vi "Logger.vi"(8 "wfm data stream":T1, 11 "file path tag":T2) -> (0 "done":bool=TRUE)   [LabVIEW 2023]
uses:
  <extravilib>/ChannelInstances/Tag-path/))Channel.ctl
  <extravilib>/ChannelInstances/Stream-a[.](wfm(dbl))/)Channel.ctl
  <extravilib>/ChannelInstances/Stream-a[.](wfm(dbl))/EndpointRead.vi
  <extravilib>/ChannelInstances/Stream-a[.](wfm(dbl))/)Channel.vi
  <resource>/ChannelSupport/_ChannelSupport/WaitIfNeeded.vi
  <extravilib>/ChannelInstances/Tag-path/EndpointRead.vi
  <vilib>/Waveform/WDTFileIO.llb/Write Waveforms to File (1D).vi
  <extravilib>/ChannelInstances/Tag-path.lvlib
  <extravilib>/ChannelInstances/Stream-a[.](wfm(dbl)).lvlib
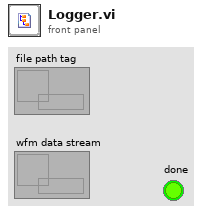
[diagram p1: front panel]
types:
  T1 = typedef "Stream-a[.](wfm(dbl)).lvlib/)Channel.ctl" = refnum<queue>
  T2 = typedef "Tag-path.lvlib/))Channel.ctl" = refnum<queue>
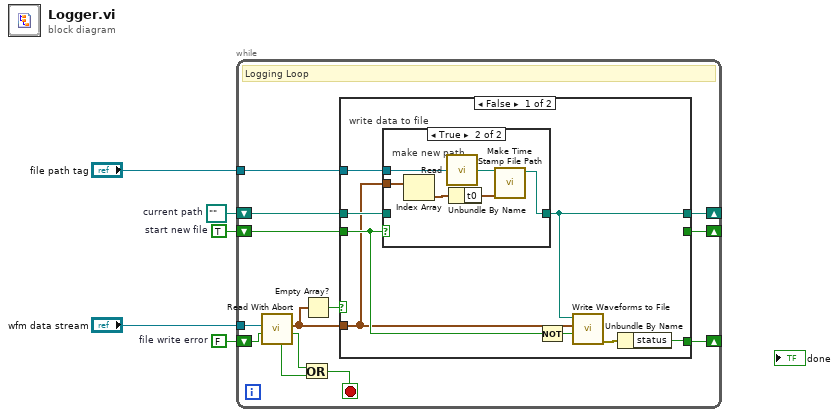
[diagram p0: block diagram]
diagram:
  w5 = FALSE  # file write error
  w4 = path ""  # current path
  w3 = TRUE  # start new file
  n1 = while {
    tunnel: "wfm data stream" -> [w18]
    tunnel: "file path tag" -> [w13]
    shift-right: [w15] -> _
    shift-left: w3 -> [w14]
    shift-right: [w12] -> _
    shift-left: w4 -> [w11]
    shift-right: [w9] -> _
    shift-left: w5 -> [w8]
    stop <- w6 stop-if-true
    # "Logging Loop"
    n2 = call <extravilib>:"Read With Abort.vi"("abort"=w8, "channel"=w18) -> ("last element?"=w16:bool, "element"=w17:waveform(dbl)[], "aborted?"=w7:bool)  [unwired: 4 in, 3 out]
    n3 = Or(x=w16, y=w7) -> (x .or. y?=w6:bool)
    n4 = Empty Array?(array=w17) -> (empty?=w10:bool)
    n5 = case shown="False" w10 {
      selector: w10 -> [_ w34]
      tunnel: w17 -> [w21 _]
      tunnel: [_ w34] -> w15
      tunnel: w14 -> [w22 _]
      tunnel: w13 -> [w25 _]
      tunnel: [w23 _] -> w12
      tunnel: w11 -> [w24 _]
      tunnel: [w19 _] -> w9
      frame False {
        # "write data to file"
        n6 = case shown="True" w22 {
          tunnel: w25 -> [_ w33]
          tunnel: w21 -> [_ w30]
          tunnel: [w27 w32] -> w23
          tunnel: w24 -> [w27 _]
          frame False {
          }
          frame True {
            # "make new path"
            n7 = Index Array(array=w30) -> (element=w31:waveform(dbl))  [unwired: 1 in]
            n8 = call <extravilib>:"Read.vi"("channel"=w33) -> ("element"=w29:path)  [unwired: 1 in, 1 out]
            n9 = Unbundle By Name(w31) -> ("t0"=w28:timestamp)
            n10 = call "Make Time Stamp File Path.vi"("t0"=w28, "base path"=w29) -> ("file path"=w32:path)  [unwired: 9 in]
          }
        }
        n11 = Not(x=w22) -> (.not. x?=w26:bool)
        n12 = call-poly <vilib>:"Write Waveforms to File.vi"("append to file? (new file:F)"=w26, "waveform array"=w21, "file path (dialog if empty)"=w23) -> ("error out"=w20:errorcluster)  [unwired: 7 in, 1 out]
        n13 = Unbundle By Name(w20) -> ("status"=w19:bool)
      }
      frame True {
        # "empty: start new file next time"
      }
    }
  }
